vi "Remove Zeros.vi"(3 "Sort by Primary Array?":bool, 4 "Primary Input Array":dbl[](array[numeric])=[80.0, 65.0, 70.0, 75.0, 25.0, 40.0, 60.0, 90.0, 50.0, 35.0, 55.0, 85.0, 20.0, 30.0, 45.0, 0.0, 0.0] format="%.2f", 5 "Slave Input Array":dbl[](array[numeric])=[287.0, 250.0, 245.0, 237.0, 8.0, 53.0, 248.0, 251.0, 159.0, 13.0, 215.0, 246.0, 9.0, 13.0, 114.0, 0.0, 0.0] format="%.2f") -> (1 "Primary Output Array":dbl[](array[numeric])=[20.0, 25.0, 30.0, 35.0, 40.0, 45.0, 50.0, 55.0, 60.0, 65.0, 70.0, 75.0, 80.0, 85.0, 90.0] format="%.2f", 2 "Slave Output Array":dbl[](array[numeric])=[9.0, 8.0, 13.0, 13.0, 53.0, 114.0, 159.0, 215.0, 248.0, 250.0, 245.0, 237.0, 287.0, 246.0, 251.0] format="%.2f")   [LabVIEW 2015]
panel:
  # "This VI meant for cleaning up plots. Takes two equal sized 1D arrays as inputs\n(typically an X and Y array). For any 0 or -999 value in the primary array, both it and its mate\nin the slave array will be removed."
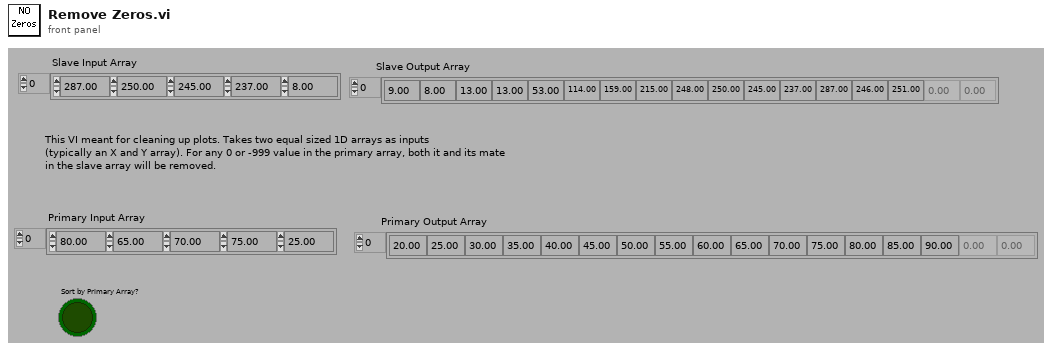
[diagram p1: front panel]
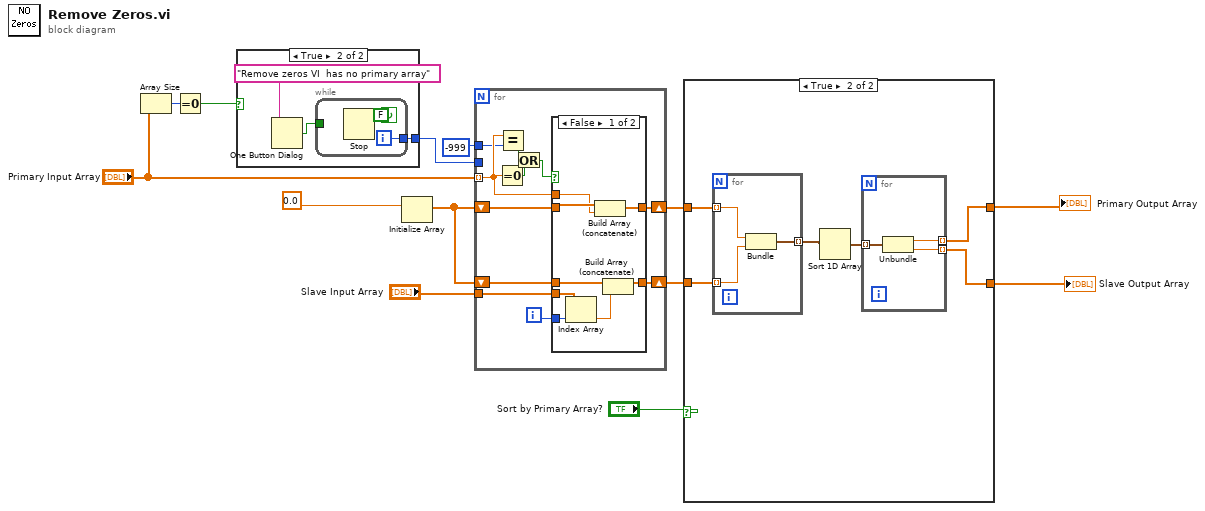
[diagram p0: block diagram]
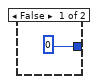
[diagram p3: hidden frame]
diagram:
  n1 = Array Size(array="Primary Input Array") -> (size(s)=w8:i32)
  n2 = Equal To 0?(x=w8) -> (x = 0?=w7:bool)
  n3 = case shown="True" w7 {
    tunnel: [0 w16] -> w6
    frame False {
    }
    frame True {
      n4 = One Button Dialog(message="Remove zeros VI  has no primary array") -> (true=w17:bool)  [unwired: 1 in]
      n5 = while {
        tunnel: [w19] -> w16
        tunnel: w17 -> [_]
        i -> [w19]
        stop <- FALSE continue-if-true
        n6 = Stop() -> ()  [unwired: 1 in]
      }
    }
  }
  n7 = Initialize Array(0.0) -> (w12:dbl[])  [unwired: 1 in]
  n8 = for {
    shift-right: [w30] -> w3
    shift-left: w12 -> [w29]
    tunnel: "Primary Input Array" -> [w21] mode=indexing
    shift-right: [w27] -> w1
    shift-left: w12 -> [w28]
    tunnel: "Slave Input Array" -> [w26]
    tunnel: -999 -> [w20]
    tunnel: w6 -> [_]
    i -> [w25]
    n9 = Equal To 0?(x=w21) -> (x = 0?=w23:bool)
    n10 = Equal?(x=w21, y=w20) -> (x = y?=w24:bool)
    n11 = Or(x=w24, y=w23) -> (x .or. y?=w22:bool)
    n12 = case shown="False" w22 {
      tunnel: [w38 w40] -> w30
      tunnel: w29 -> [w37 w40]
      tunnel: w21 -> [w36 _]
      tunnel: w28 -> [w35 w39]
      tunnel: [w34 w39] -> w27
      tunnel: w26 -> [w32 _]
      tunnel: w25 -> [w33 _]
      frame False {
        n13 = Index Array(array=w32, index=w33) -> (element=w31:dbl)
        n14 = Build Array (concatenate)(w37, w36) -> (w38:dbl[])
        n15 = Build Array (concatenate)(w35, w31) -> (w34:dbl[])
      }
      frame True {
      }
    }
  }
  n16 = case shown="True" "Sort by Primary Array?" {
    tunnel: [w42 w44] -> w4
    tunnel: w3 -> [w42 w48]
    tunnel: [w41 w43] -> w2
    tunnel: w1 -> [w41 w47]
    frame False {
    }
    frame True {
      n17 = for {
        tunnel: w48 -> [w54] mode=indexing
        tunnel: w47 -> [w53] mode=indexing
        tunnel: [w52] -> w46 mode=indexing
        n18 = Bundle(w54, w53) -> (w52:cluster{dbl, dbl})  [unwired: 1 in]
      }
      n19 = Sort 1D Array(array=w46) -> (sorted array=w45:cluster{dbl, dbl}[])
      n20 = for {
        tunnel: w45 -> [w51] mode=indexing
        tunnel: [w50] -> w44 mode=indexing
        tunnel: [w49] -> w43 mode=indexing
        n21 = Unbundle(w51) -> (w50:dbl, w49:dbl)
      }
    }
  }
  "Primary Output Array" <- w4
  "Slave Output Array" <- w2
